vi "Save Lockin Metadata.vi"(8 "error in (no error)":errorcluster, 11 "Red Pitaya Digitizer in":refnum<class "Red Pitaya Digitizer.lvclass">) -> (0 "error out":errorcluster, 3 "Red Pitaya Digitizer out":refnum<class "Red Pitaya Digitizer.lvclass">)   [LabVIEW 2024, in "Red Pitaya Digitizer.lvclass"]
uses:
  Red Pitaya Digitizer.lvclass
  Red Pitaya Digitizer.lvclass/Red Pitaya Digitizer.ctl
  RP Core/RP Instrument/RP Instrument.lvclass
  Instruments/Pulse Driver/Lockin Digitizer Driver/Lockin Digitizer Driver.lvclass
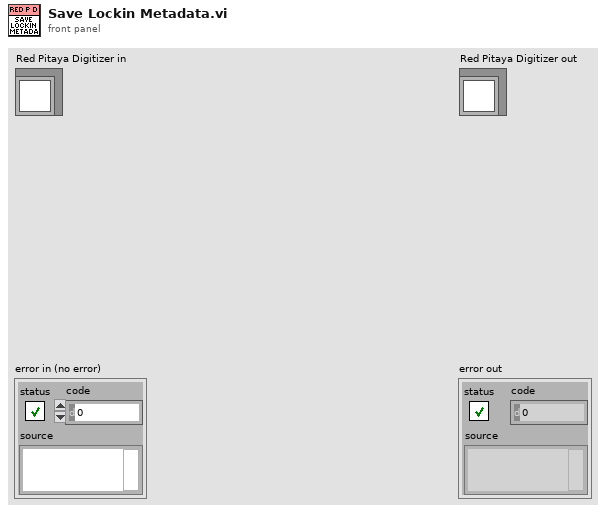
[diagram p1: front panel]
types:
  T1 = typedef "Lockin Digitizer Configuration.ctl" = cluster{"Post-trigger delay":dbl, "Post-trigger duration":dbl, "Rate":dbl, "Ranges":dbl[], "Re-name channels":string[], "Active channels":string, "External\nclock":bool, "Frequencies":dbl[], "Monitor time\nconstant":dbl, "Output \namplitudes":dbl[], "Input\nchannles":string[], "Sync":bool, "Lock-in input channel phases":dbl[]}
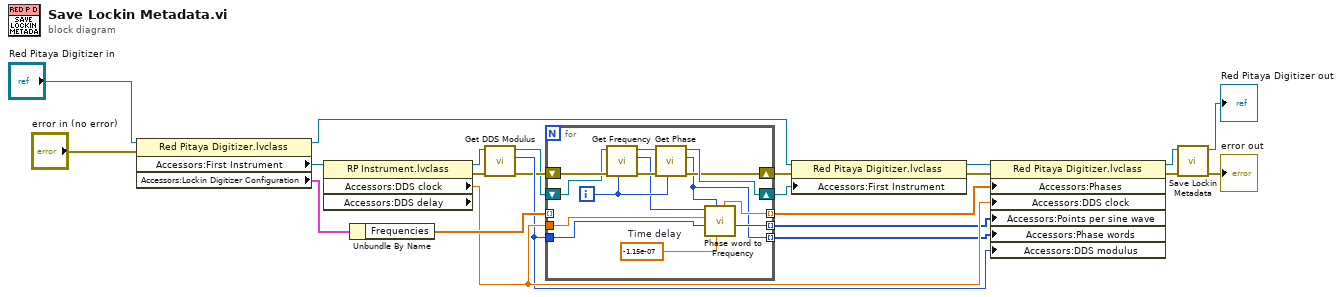
[diagram p0: block diagram]
diagram:
  n1 = property class="Red Pitaya Digitizer.lvclass"(reference="Red Pitaya Digitizer in", error in="error in (no error)") -> (reference out=w17:refnum<class "Red Pitaya Digitizer.lvclass">, "Accessors:First Instrument"=w12:refnum<class "RP Instrument.lvclass">, "Accessors:Lockin Digitizer Configuration"=w11:T1)  [unwired: 1 out]
  n2 = property class="RP Instrument.lvclass" props=["Accessors:DDS clock", "Accessors:DDS delay"](reference=w12) -> (reference out=w8:refnum<class "RP Instrument.lvclass">, error out=w9:errorcluster, "Accessors:DDS clock"=w10:dbl)  [unwired: 1 in, 1 out]
  n3 = Unbundle By Name(w11) -> ("Frequencies"=w19:dbl[])
  n4 = call-dynamic "Get DDS Modulus.vi"("error in (no error)"=w9, "RP Instrument in"=w8) -> ("error out"=w4:errorcluster, "DDS modulus"=w5:i64, "RP Instrument out"=w3:refnum<class "RP Instrument.lvclass">)  [unwired: 7 in]
  n5 = for {
    tunnel: w19 -> [_] mode=indexing
    shift-right: [w30] -> w2
    shift-left: w3 -> [w36]
    tunnel: [w31] -> w18 mode=indexing
    shift-right: [w29] -> w1
    shift-left: w4 -> [w37]
    tunnel: w10 -> [w28]
    tunnel: w5 -> [w27]
    tunnel: [w25] -> w7 mode=indexing
    tunnel: [w24] -> w6 mode=indexing
    i -> [w33]
    w26 = -1.15e-07  # Time delay
    n6 = call-dynamic "Get Frequency.vi"("Output channel"=w33, "error in (no error)"=w37, "RP Instrument in"=w36) -> ("error out"=w35:errorcluster, "Frequency"=w32:u32, "RP Instrument out"=w34:refnum<class "RP Instrument.lvclass">)  [unwired: 6 in]
    n7 = call-dynamic "Get Phase.vi"("Output channel"=w33, "error in (no error)"=w35, "RP Instrument in"=w34) -> ("error out"=w29:errorcluster, "Phase"=w24:u32, "RP Instrument out"=w30:refnum<class "RP Instrument.lvclass">)  [unwired: 6 in]
    n8 = call "Phase word to Frequency.vi"("Time delay"=w26, "Phase word"=w24, "DDS modulus"=w27, "DDS clock"=w28, "Frequency word"=w32) -> ("Points per sine wave"=w25:u64, "Phase"=w31:dbl)  [unwired: 3 in, 2 out]
  }
  n9 = property class="Red Pitaya Digitizer.lvclass"(reference=w17, error in=w1, "Accessors:First Instrument"=w2) -> (reference out=w16:refnum<class "Red Pitaya Digitizer.lvclass">, error out=w15:errorcluster)
  n10 = property class="Red Pitaya Digitizer.lvclass"(reference=w16, error in=w15, "Accessors:Phases"=w18, "Accessors:DDS clock"=w10, "Accessors:Points per sine wave"=w7, "Accessors:Phase words"=w6, "Accessors:DDS modulus"=w5) -> (reference out=w13:refnum<class "Red Pitaya Digitizer.lvclass">, error out=w14:errorcluster)
  n11 = call-parent "Save Lockin Metadata.vi"("error in (no error)"=w14, "Lockin Digitizer Driver in"=w13) -> ("error out"=→"error out":errorcluster, "Lockin Digitizer Driver out"=→"Red Pitaya Digitizer out":refnum<class "Red Pitaya Digitizer.lvclass">)  [unwired: 8 in]
